vi "Start.vi"(8 "error in":errorcluster, 11 "gRPC XNET Read Raw CAN Frame Strategy in":refnum<class "gRPC XNET Read Raw CAN Frame Strategy.lvclass">) -> (0 "error out":errorcluster, 3 "gRPC XNET Read Raw CAN Frame Strategy out":refnum<class "gRPC XNET Read Raw CAN Frame Strategy.lvclass">)   [LabVIEW 2024, in "gRPC XNET Read Raw CAN Frame Strategy.lvclass"]
uses:
  gRPC XNET Read Raw CAN Frame Strategy.lvclass
  grpc-xnet/grpc-xnet_client/RPC Messages/nixnet_grpc_StartRequest_scope_enum/nixnet_grpc_StartRequest_scope_enum.lvclass
  grpc-xnet/grpc-xnet_client/RPC Messages/nixnet_grpc_StartRequest_scope_enum/nixnet_grpc_StartRequest_scope_enum.lvclass/nixnet_grpc_StartRequest_scope_enum.ctl
  gRPC XNET Read Raw CAN Frame Strategy.lvclass/gRPC XNET Read Raw CAN Frame Strategy.ctl
  grpc-xnet/grpc-xnet_client/grpc-xnet_client.lvlib
  grpc-xnet/grpc-xnet_client/RPC Messages/nixnet_grpc_StartStopScope.ctl
  grpc-xnet/grpc-xnet_client/RPC Messages/nidevice_grpc_Session.ctl
  grpc-xnet/grpc-xnet_client/RPC Messages/nixnet_grpc_StartRequest.ctl
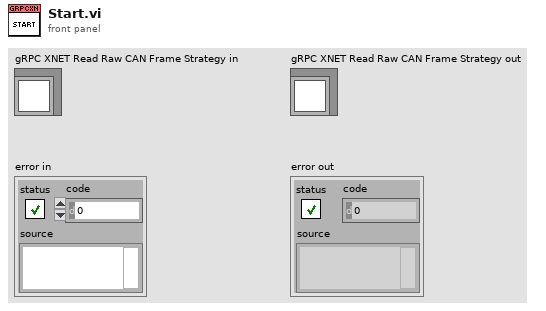
[diagram p1: front panel]
types:
  T1 = typedef "grpc-xnet_client.lvlib/nixnet_grpc_StartRequest.ctl" = cluster{"session":T2, "nixnet_grpc_StartRequest_scope_enum":refnum<class "nixnet_grpc_StartRequest_scope_enum.lvclass">}
  T2 = typedef "grpc-xnet_client.lvlib/nidevice_grpc_Session.ctl" = cluster{"name":string}
  T3 = typedef "grpc-xnet_client.lvlib/nixnet_grpc_StartStopScope.ctl" = enum32{"START_STOP_SCOPE_NORMAL", "START_STOP_SCOPE_SESSION_ONLY", "START_STOP_SCOPE_INTERFACE_ONLY", "START_STOP_SCOPE_SESSION_ONLY_BLOCKING"}
  T4 = typedef "grpc-lvsupport-release.lvlib/grpcId.ctl" = u64
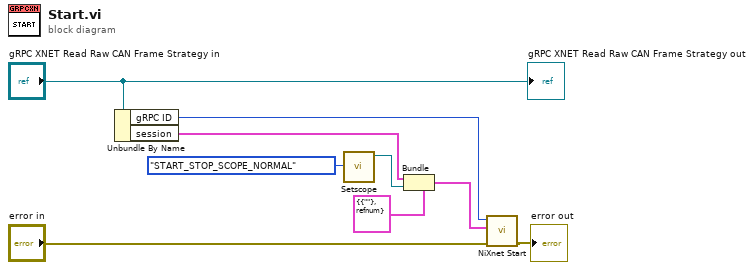
[diagram p0: block diagram]
diagram:
  n1 = Unbundle By Name("gRPC XNET Read Raw CAN Frame Strategy in") -> ("gRPC ID"=w7:T4, "session"=w5:T2)
  n2 = call "Setscope.vi"("Set_Val"=nixnet_grpc_StartStopScope."START_STOP_SCOPE_NORMAL") -> ("OneOfTemplate out"=w4:refnum<class "nixnet_grpc_StartRequest_scope_enum.lvclass">)  [unwired: 9 in, 1 out]
  n3 = Bundle(cluster=T1 {"session"={"name"=""}, "nixnet_grpc_StartRequest_scope_enum"=refnum} ("Request Data"), "session"=w5, "nixnet_grpc_StartRequest_scope_enum"=w4) -> (w2:T1)
  n4 = call "NiXnet Start.vi"("error in"="error in", "Request Data"=w2, "gRPC ID"=w7) -> ("error out"=→"error out":errorcluster)  [unwired: 6 in, 2 out]
  "gRPC XNET Read Raw CAN Frame Strategy out" <- "gRPC XNET Read Raw CAN Frame Strategy in"
